vi "Step Convert Record To jsRecord.vi"(0 "Making Copy? (f)":bool, 3 "Descriptions":string[](array[string]), 4 "Test_IDs":string[](array[string]), 5 "Step Record":T1) -> (2 "STEP jsRecord":T2)   [LabVIEW 2011]
uses:
  Step jsRecord.ctl
  Step Record.ctl
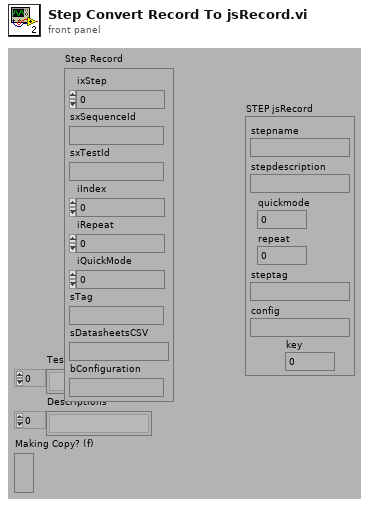
[diagram p1: front panel]
types:
  T1 = typedef "Step Record.ctl" = cluster{"ixStep":i32, "sxSequenceId":string, "sxTestId":string, "iIndex":i32, "iRepeat":i32, "iQuickMode":i32, "sTag":string, "sDatasheetsCSV":string, "bConfiguration":string}
  T2 = typedef "Step jsRecord.ctl" = cluster{"stepname":string, "stepdescription":string, "quickmode":i32, "repeat":i32, "steptag":string, "config":string, "key":i32}
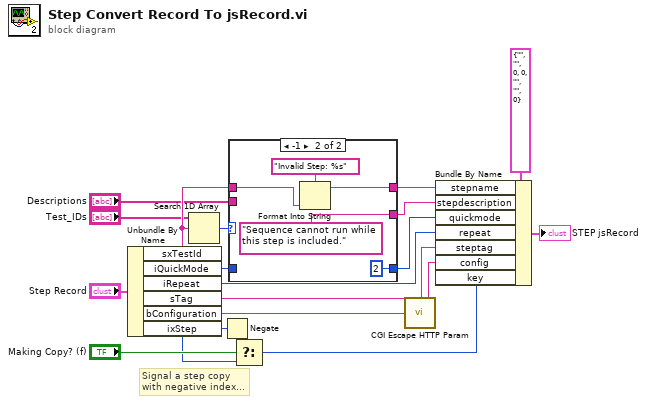
[diagram p0: block diagram]
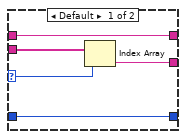
[diagram p2: hidden frame]
diagram:
  # "Signal a step copy\nwith negative index..."
  n1 = Unbundle By Name("Step Record") -> ("sxTestId"=w18:string, "iQuickMode"=w12:i32, "iRepeat"=w14:i32, "sTag"=w13:string, "bConfiguration"=w2:string, "ixStep"=w4:i32)
  n2 = Search 1D Array(1D array="Test_IDs", element=w18) -> (index of element=w3:i32)  [unwired: 1 out]
  n3 = Negate(x=w4) -> (-x=w10:i32)
  n4 = case shown="-1" w3 {
    selector: w3 -> [w20 _]
    tunnel: w18 -> [w24 w28]
    tunnel: [w24 w27] -> w17
    tunnel: [w22 "Sequence cannot run while this step is included."] -> w16
    tunnel: "Descriptions" -> [w23 _]
    tunnel: [w21 2] -> w15
    tunnel: w12 -> [w21 _]
    frame Default {
      n5 = Index Array(array=w23, index=w20) -> (element=w22:string)
    }
    frame -1 {
      n6 = Format Into String(format string="Invalid Step: %s", w28) -> (resulting string=w27:string)  [unwired: 2 in, 1 out]
    }
  }
  n7 = Select(t=w10, s="Making Copy? (f)", f=w4) -> (s? t:f=w11:i32)
  n8 = call <vilib>:"CGI Escape HTTP Param.vi"("string"=w2) -> ("url-encoded string"=w1:string)
  n9 = Bundle By Name(cluster=T2 {"stepname"="", "stepdescription"="", "quickmode"=0, "repeat"=0, "steptag"="", "config"="", "key"=0} ("STEP javascript object"), "stepname"=w17, "stepdescription"=w16, "quickmode"=w15, "repeat"=w14, "steptag"=w13, "config"=w1, "key"=w11) -> (→"STEP jsRecord":T2)
